vi "finishTableWith2ndStrikerPlay.vi"(10 "Game":refnum<class "Game.lvclass">, 11 "TableWith2ndStrikerPlay in":refnum<class "TableWith2ndStrikerPlay.lvclass">) -> (2 "finishTableWith2ndStriker?":bool, 3 "TableWith2ndStrikerPlay out":refnum<class "TableWith2ndStrikerPlay.lvclass">)   [LabVIEW 2020, in "TableWith2ndStrikerPlay.lvclass"]
uses:
  TableWith2ndStrikerPlay.lvclass
  Game_class/Game.lvclass
  Referee_class/command_interpreted.ctl
  Game_class/Game.lvclass/Game.ctl
  Referee_class/Referee.lvclass/Referee.ctl
  Events_class/Events.lvclass/Events.ctl
  Team_class/Team.lvclass/Team.ctl
  Game_class/Read EventsRef.vi
  Game_class/Read BallRef.vi
  Game_class/Read OffensiveTeam.vi
  Team_class/Read RobotRef.vi
  Events_class/Read touch.vi
  Events_class/Read id_touch.vi
  Events_class/Read ball_out.vi
  Game_class/Read Referee.vi
  Referee_class/Read command_interpreted.vi
  Ally_class/Ally.lvclass
  Referee_class/Referee.lvclass
  Events_class/Events.lvclass
  Ball_class/Ball.lvclass
  Robot_class/Robot.lvclass
  Play_class/Play.lvclass
panel:
  out "error out":errorcluster
  in  "error in (no error)":errorcluster
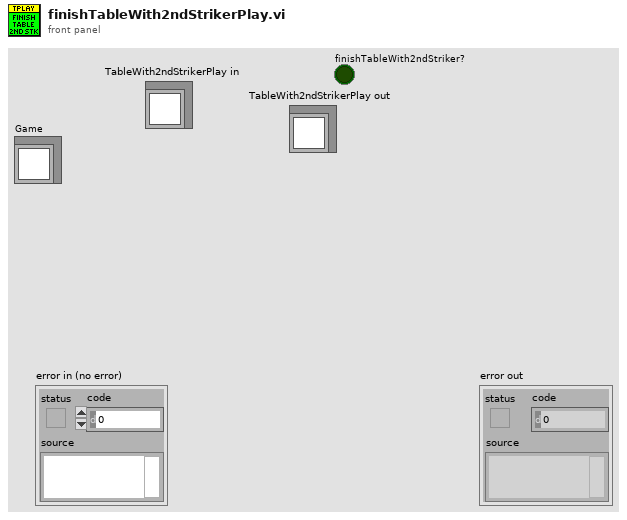
[diagram p1: front panel]
types:
  T1 = typedef "command_interpreted.ctl" = enum16{"Goal Ally", "Goal Enemy", "Ball Placement Enemy", "Ball Placement Ally", "Normal Half Time", "Extra Time  Break", "Extra Half Time", "None", "Post Game", "PKA Normal Start", "Prepare Kickoff Ally", "PKE Normal Start", "Prepare Kickoff Enemy", "Force Start", "Halt", "Timeout", "Prepare Penalty Ally", "Prepare Penalty Enemy", "PPA NormalStart", "PPE Normal Start", "Indirect Free Ally", "Direct Free Enemy", "Direct Free Ally", "Indirect Free Enemy", "Stop"}
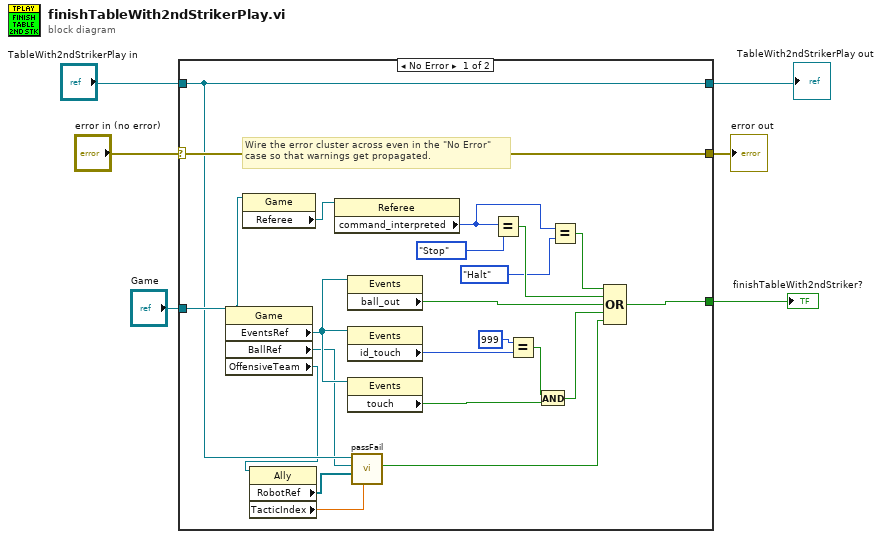
[diagram p0: block diagram]
diagram:
  n1 = case shown="No Error" "error in (no error)" {
    selector: "error in (no error)" -> [w28 w30]
    tunnel: [w28 w30] -> w5
    tunnel: [w12 w29] -> w1
    tunnel: "TableWith2ndStrikerPlay in" -> [w12 w29]
    tunnel: [w19 _] -> w4
    tunnel: "Game" -> [w18 _]
    frame No Error {
      # "Wire the error cluster across even in the \"No Error\"\ncase so that warnings get propagated."
      n2 = property class="Game"(reference=w18) -> ("EventsRef"=w27:refnum<class "Events.lvclass">, "BallRef"=w9:refnum<class "Ball.lvclass">, "OffensiveTeam"=w11:refnum<class "Ally.lvclass">)  [unwired: 1 in, 2 out]
      n3 = property class="Game"(reference=w18) -> ("Referee"=w21:refnum<class "Referee.lvclass">)  [unwired: 1 in, 2 out]
      n4 = property class="Ally"(reference=w11) -> ("RobotRef"=w10:refnum<class "Robot.lvclass">[], "TacticIndex"=w7:dbl)  [unwired: 1 in, 2 out]
      n5 = property class="Referee"(reference=w21) -> ("command_interpreted"=w15:T1)  [unwired: 1 in, 2 out]
      n6 = property class="Events"(reference=w27) -> ("ball_out"=w24:bool)  [unwired: 1 in, 2 out]
      n7 = property class="Events"(reference=w27) -> ("id_touch"=w25:i32)  [unwired: 1 in, 2 out]
      n8 = property class="Events"(reference=w27) -> ("touch"=w20:bool)  [unwired: 1 in, 2 out]
      n9 = call "passFail.vi"("TacticIndex"=w7, "Offensive Robots"=w10, "Ball"=w9, "Play in"=w12) -> ("PassFail?"=w8:bool)  [unwired: 5 in, 2 out]
      n10 = Equal?(x=w15, y=command_interpreted."Stop") -> (x = y?=w16:bool)
      n11 = Equal?(x=999 ("id_touch"), y=w25) -> (x = y?=w23:bool)
      n12 = And(x=w23, y=w20) -> (x .and. y?=w22:bool)
      n13 = Equal?(x=w15, y=command_interpreted."Halt") -> (x = y?=w13:bool)
      n14 = Compound Arithmetic op=OR(w13, w16, w24, w22, w8) -> (w19:bool)
    }
    frame Error {
    }
  }
  "error out" <- w5
  "finishTableWith2ndStriker?" <- w4
  "TableWith2ndStrikerPlay out" <- w1
